vi "Measurement.Init.vi"(8 "error in (no error)":errorcluster, 10 "timeout (5000 ms)":i32=5000, 11 "Measurement.PhotocurrentMapping in":refnum<class "Measurement.PhotocurrentMapping.lvclass">) -> (0 "error out":errorcluster, 1 "Dependencies Results":bool[](array[boolean]), 2 "Result":bool, 3 "Measurement.PhotocurrentMapping out":refnum<class "Measurement.PhotocurrentMapping.lvclass">)   [LabVIEW 2017, in "Measurement.PhotocurrentMapping.lvclass"]
uses:
  Measurement.PhotocurrentMapping.lvclass
  XYStage/XYStage.lvclass
  D:/upwork/Laser Measurement Tool/Laser/project/Subsystems/Device/Device.lvclass
  SMU/SMU.lvclass
  LIA/LIA.lvclass
  Device/Device.lvclass
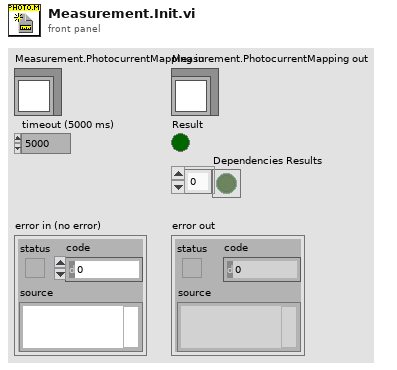
[diagram p1: front panel]
types:
  T1 = typedef "Measurement.PhotocurrentMapping.lvclass/Configuration--Cluster.ctl" = cluster{"Measurement.Type":T2, "Hardware":T3, "Measurement":T10}
  T2 = typedef "Measurement.lvclass/Measurement.Type--Enum.ctl" = enum16{"Free", "I/V Curve", "Wavelength sweeping", "Photocurrent mapping"}
  T3 = typedef "Measurement.PhotocurrentMapping.lvclass/Configuration.Hardware--Cluster.ctl" = cluster{"SMU":T4, "LIA":T6, "XYStage":T8}
  T4 = typedef "Measurement.lvclass/Configuration.SMU--Cluster.ctl" = cluster{"Enable":bool, "SMU Model":string, "Configuration":T5}
  T5 = typedef "SMU.lvclass/Configuration--Cluster.ctl" = cluster{"VISA Resource":string, "Channel":string}
  T6 = typedef "Measurement.lvclass/Configuration.LIA--Cluster.ctl" = cluster{"Enable":bool, "LIA Model":string, "Configuration":T7}
  T7 = typedef "LIA.lvclass/Configuration--Cluster.ctl" = cluster{"VISA Resource":string}
  T8 = typedef "Measurement.lvclass/Configuration.XYStage--Cluster.ctl" = cluster{"Enable":bool, "XYStage Model":string, "Configuration":T9}
  T9 = typedef "XYStage.lvclass/Configuration--Cluster.ctl" = cluster{"Serial Number":string, "X Axis":string, "Y Axis":string, "Real-World Units":string, "Counts per Unit":u32}
  T10 = typedef "Measurement.PhotocurrentMapping.lvclass/Configuration.Measurement--Cluster.ctl" = cluster{"X":T11, "Y":T11, "Accumulation":u16}
  T11 = typedef "Measurement.PhotocurrentMapping.lvclass/Configuration.Axis--Cluster.ctl" = cluster{"Start, units":dbl, "Stop, units":dbl, "Step, units":dbl}
  T12 = typedef "Measurement.PhotocurrentMapping.lvclass/Dependencies--Cluster.ctl" = cluster{"SMU":refnum<class "SMU.lvclass">, "LIA":refnum<class "LIA.lvclass">, "XYStage":refnum<class "XYStage.lvclass">}
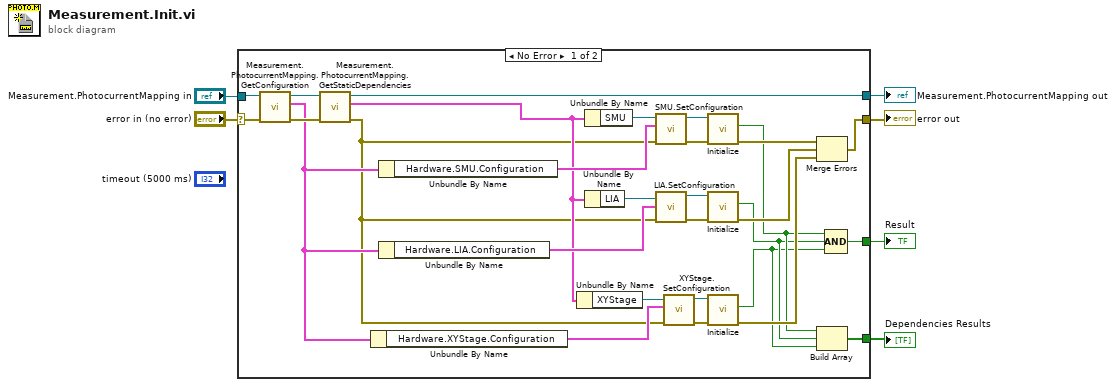
[diagram p0: block diagram]
diagram:
  n1 = case shown="No Error" "error in (no error)" {
    selector: "error in (no error)" -> [w34 w36]
    tunnel: "Measurement.PhotocurrentMapping in" -> [w35 w37]
    tunnel: [w15 w37] -> w4
    tunnel: [w14 w36] -> w3
    tunnel: [w13 _] -> w1
    tunnel: [w12 _] -> w2
    frame No Error {
      n2 = call "Measurement.PhotocurrentMapping.GetConfiguration.vi"("error in (no error)"=w34, "Measurement.PhotocurrentMapping"=w35) -> ("error out"=w32:errorcluster, "Configuration"=w17:T1, "Measurement.PhotocurrentMapping out"=w33:refnum<class "Measurement.PhotocurrentMapping.lvclass">)  [unwired: 7 in]
      n3 = call "Measurement.PhotocurrentMapping.GetStaticDependencies.vi"("error in (no error)"=w32, "Measurement.PhotocurrentMapping in"=w33) -> ("error out"=w8:errorcluster, "Dependencies"=w16:T12, "Measurement.PhotocurrentMapping out"=w15:refnum<class "Measurement.PhotocurrentMapping.lvclass">)  [unwired: 7 in]
      n4 = Unbundle By Name(w17) -> ("Hardware.XYStage.Configuration"=w9:T9)
      n5 = Unbundle By Name(w17) -> ("Hardware.SMU.Configuration"=w30:T5)
      n6 = Unbundle By Name(w17) -> ("Hardware.LIA.Configuration"=w25:T7)
      n7 = Unbundle By Name(w16) -> ("XYStage"=w11:refnum<class "XYStage.lvclass">)
      n8 = Unbundle By Name(w16) -> ("SMU"=w31:refnum<class "SMU.lvclass">)
      n9 = Unbundle By Name(w16) -> ("LIA"=w26:refnum<class "LIA.lvclass">)
      n10 = call "SMU.SetConfiguration.vi"("error in (no error)"=w8, "Configuration"=w30, "SMU"=w31) -> ("error out"=w28:errorcluster, "SMU out"=w29:refnum<class "SMU.lvclass">)  [unwired: 7 in]
      n11 = call "LIA.SetConfiguration.vi"("error in (no error)"=w8, "Configuration"=w25, "LIA"=w26) -> ("error out"=w24:errorcluster, "LIA out"=w23:refnum<class "LIA.lvclass">)  [unwired: 7 in]
      n12 = call "XYStage.SetConfiguration.vi"("error in (no error)"=w8, "Configuration"=w9, "XYStage"=w11) -> ("error out"=w7:errorcluster, "XYStage out"=w10:refnum<class "XYStage.lvclass">)  [unwired: 7 in]
      n13 = call "Initialize.vi"("error in (no error)"=w28, "Device in"=w29) -> ("error out"=w27:errorcluster, "Result"=w20:bool)  [unwired: 7 in, 1 out]
      n14 = call "Initialize.vi"("error in (no error)"=w24, "Device in"=w23) -> ("error out"=w22:errorcluster, "Result"=w19:bool)  [unwired: 7 in, 1 out]
      n15 = call "Initialize.vi"("error in (no error)"=w7, "Device in"=w10) -> ("error out"=w21:errorcluster, "Result"=w18:bool)  [unwired: 7 in, 1 out]
      n16 = Merge Errors(w27, w22, w21) -> (w14:errorcluster)
      n17 = Build Array(w20, w19, w18) -> (w12:bool[])
      n18 = Compound Arithmetic op=AND(w20, w19, w18) -> (w13:bool)
    }
    frame Error {
    }
  }
  "error out" <- w3
  "Measurement.PhotocurrentMapping out" <- w4
  "Result" <- w1
  "Dependencies Results" <- w2
